vi "mainOCR.vi"() -> ()   [LabVIEW 2025]
uses:
  ocr/ocr.lvclass
  ocr/TextDecRecResult2L.ctl
  ocr/ocrParameters.ctl
panel:
  out "loadImgSucc":string
  out "succ 2":i32
  in  "Default Parameters":bool
  in  "device":enum16{"CPU", "GPU0"}(ring)
  out "InitRecDec Success":string
  out "SetDevice":string
  in  "ocrParameters":T1={"targetSize"=1088, "expandRatio "=1.12, "padPixels "=10, "binThresh"=0.3, "txt_score_thresh"=0.25, "minArea"=12, "cropMargin"=5, "binSize"=32}
  in  "PathImage":path=path "D:/Test/dllTest/images_2"
  out "Image":T2(plugin-control)
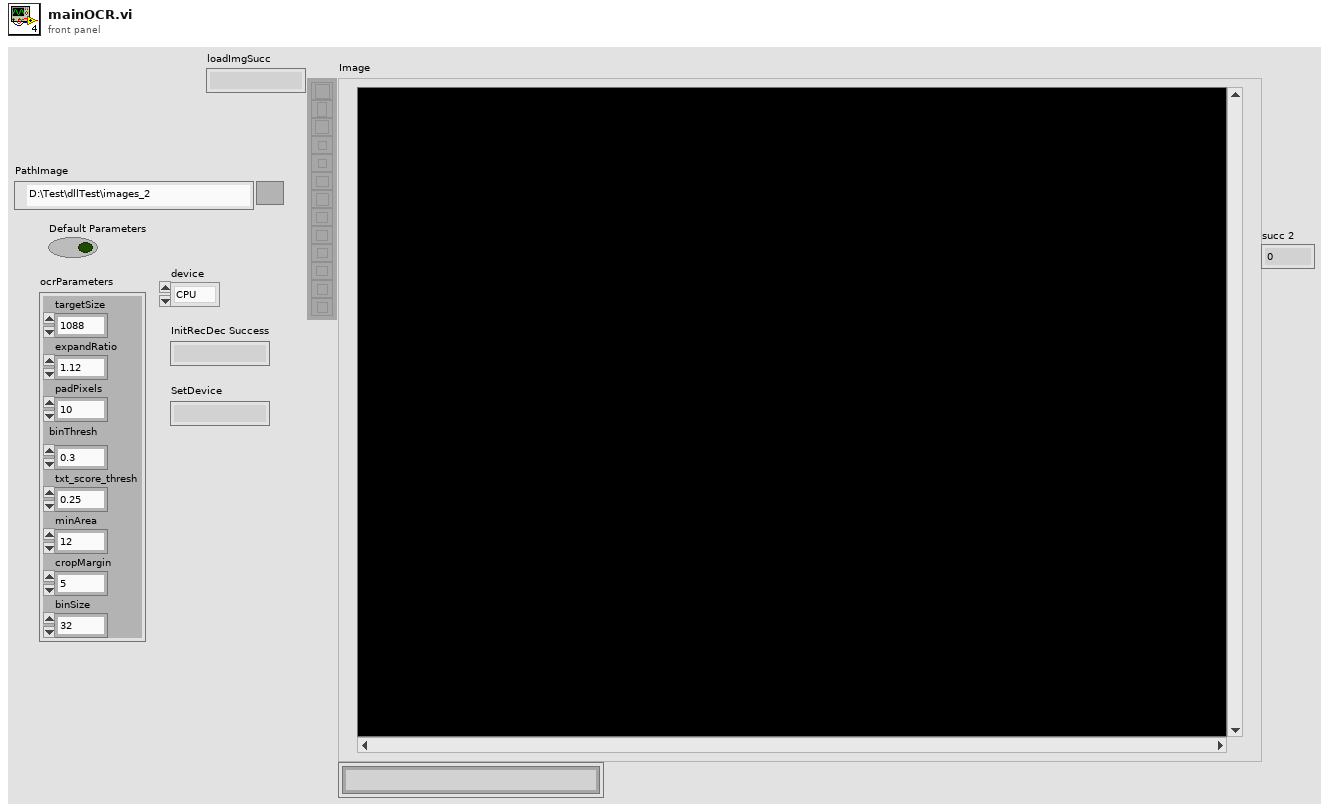
[diagram p1: front panel]
types:
  T1 = typedef "adsToolkit.lvlib/ocr.lvclass/ocrParameters.ctl" = cluster{"targetSize":i32, "expandRatio ":sgl, "padPixels ":i32, "binThresh":sgl, "txt_score_thresh":sgl, "minArea":i32, "cropMargin":i32, "binSize":i32}
  T2 = typedef "IMAQ Image.ctl" = refnum<image>
  T3 = typedef "adsToolkit.lvlib/ocr.lvclass/TextDecRecResult2L.ctl" = cluster{"imgIdx":i32, "TLx":i32, "TLy":i32, "BRx":i32, "BRy":i32, "angle":sgl, "txtLen":i32}
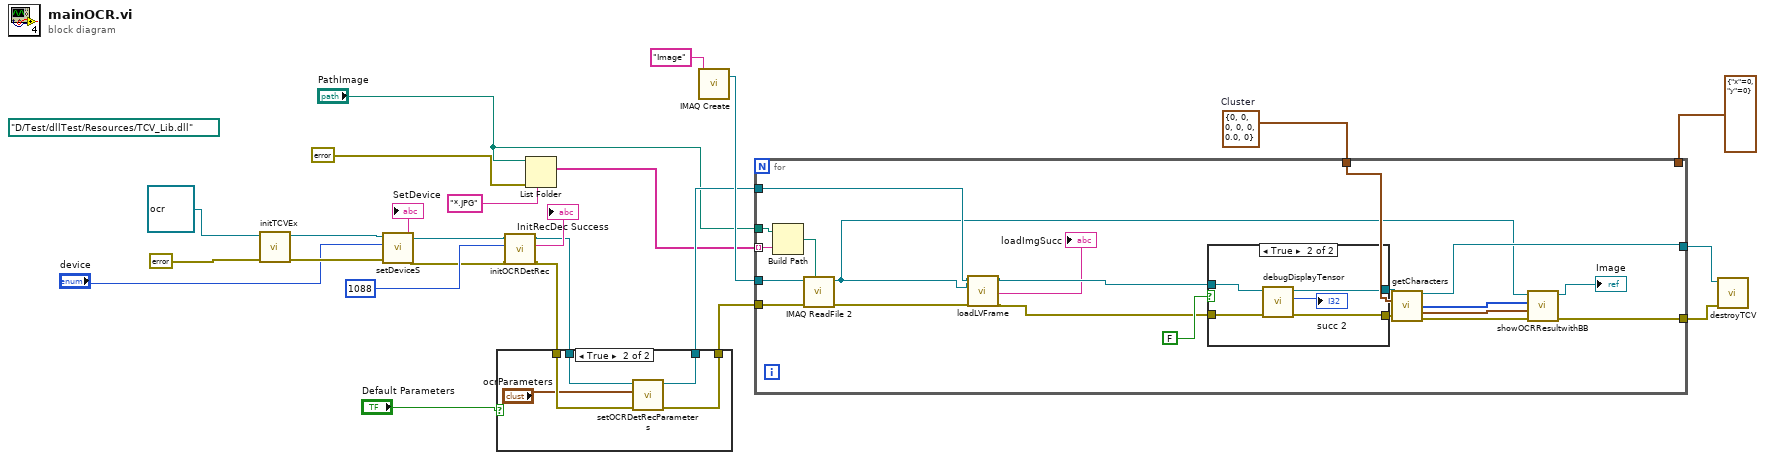
[diagram p0: block diagram]
diagram:
  w9 = T3 {"imgIdx"=0, "TLx"=0, "TLy"=0, "BRx"=0, "BRy"=0, "angle"=0.0, "txtLen"=0}  # Cluster
  (unwired) path "D:/Test/dllTest/Resources/TCV_Lib.dll" ("path in")
  n1 = call-dynamic "initTCVEx.vi"("error in (no error)"=errorcluster {"status"=FALSE, "code"=0, "source"=""}, "adsBase in"=refnum<class "ocr.lvclass"> refnum ("ocr in")) -> ("error out"=w18:errorcluster, "adsBase out"=w19:refnum<class "ocr.lvclass">)  [unwired: 8 in]
  n2 = call-dynamic "setDeviceS.vi"("error in (no error)"=w18, "devices"="device", "adsBase in"=w19) -> ("error out"=w4:errorcluster, "SetDevice"=→"SetDevice":string, "adsBase out"=w5:refnum<class "ocr.lvclass">)  [unwired: 6 in]
  n3 = call-dynamic "initOCRDetRec.vi"("error in (no error)"=w4, "targetSize"=1088, "adsBase in"=w5) -> ("error out"=w2:errorcluster, "InitRecDec Success"=→"InitRecDec Success":string, "adsBase out"=w1:refnum<class "ocr.lvclass">)  [unwired: 5 in, 1 out]
  n4 = case shown="True" "Default Parameters" {
    tunnel: w1 -> [w27 w32]
    tunnel: [w27 w31] -> w17
    tunnel: w2 -> [w26 w30]
    tunnel: [w26 w29] -> w16
    frame False {
    }
    frame True {
      n5 = call-dynamic "setOCRDetRecParameters.vi"("error in (no error)"=w30, "ocrParameters"="ocrParameters", "adsBase in"=w32) -> ("error out"=w29:errorcluster, "adsBase out"=w31:refnum<class "ocr.lvclass">)  [unwired: 5 in, 2 out]
    }
  }
  n6 = List Folder(path="PathImage", pattern="*.JPG", error in=errorcluster {"status"=FALSE, "code"=0, "source"=""}) -> (filenames=w12:string[])  [unwired: 1 in, 3 out]
  n7 = call "IMAQ Create"("Image Name"="Image") -> ("New Image"=w24:T2)  [unwired: 4 in, 1 out]
  n8 = for {
    tunnel: "PathImage" -> [w53]
    tunnel: w24 -> [w51]
    tunnel: cluster{"x":i32, "y":i32} {"x"=0, "y"=0} -> [_]
    tunnel: w17 -> [w38]
    tunnel: w9 -> [w50]
    tunnel: w16 -> [w49]
    tunnel: w12 -> [w48] mode=indexing
    tunnel: [w47] -> w10
    tunnel: [w42] -> w8
    n9 = Build Path(base path=w53, name or relative path=w48) -> (appended path=w52:path)
    n10 = call "IMAQ ReadFile 2"("File Path"=w52, "error in (no error)"=w49, "Image"=w51) -> ("error out"=w36:errorcluster, "Image Out"=w37:T2)  [unwired: 4 in, 3 out]
    n11 = call-dynamic "loadLVFrame.vi"("adsBase in"=w38, "Image"=w37, "error in (no error)"=w36) -> ("adsBase out"=w35:refnum<class "ocr.lvclass">, "loadImgSucc"=→"loadImgSucc":string, "error out"=w33:errorcluster)  [unwired: 13 in, 1 out]
    n12 = case shown="True" FALSE {
      tunnel: [w55 w60] -> w46
      tunnel: [w54 w59] -> w45
      tunnel: w35 -> [w55 w57]
      tunnel: w33 -> [w54 w56]
      frame False {
      }
      frame True {
        n13 = call-dynamic "debugDisplayTensor.vi"("error in (no error)"=w56, "adsBase in"=w57) -> ("error out"=w59:errorcluster, "succ"=→"succ 2":i32, "adsBase out"=w60:refnum<class "ocr.lvclass">)  [unwired: 6 in, 1 out]
      }
    }
    n14 = call-dynamic "getCharacters.vi"("adsBase in"=w46, "Cluster"=w50, "error in (no error)"=w45) -> ("adsBase out"=w47:refnum<class "ocr.lvclass">, "chars"=w39:u8[], "TextDecRecResult2L"=w40:T3[], "error out"=w41:errorcluster)  [unwired: 8 in, 1 out]
    n15 = call "showOCRResultwithBB.vi"("error in"=w41, "Array"=w40, "chars"=w39, "Image in"=w37) -> ("error out"=w42:errorcluster, "Image out"=→"Image":T2)  [unwired: 4 in]
  }
  n16 = call-dynamic "destroyTCV.vi"("error in (no error)"=w8, "adsBase in"=w10) -> ()  [unwired: 8 in, 2 out]
